vi "Actor Core.vi"(8 "error in":errorcluster, 11 "UDP_transmitter in":refnum<class "UDP_transmitter.lvclass">) -> (0 "error out":errorcluster, 3 "Actor out":refnum<class "Actor.lvclass">)   [LabVIEW 2025, in "UDP_transmitter.lvlib" / "UDP_transmitter.lvclass"]
doc: "(<B>Filename</B>: Actor Framework.lvlib:Actor.lvclass:Actor Core.vi)\n\nReceives messages to the actor, reacts to them, and initiates any error handling that may shut the actor down.\n\nDescendant classes may override this VI to append parallel tasks for the actor to complete while it handles messages. Overrides use the Call Parent Class Method node."
uses:
  UDP_transmitter.lvclass
  C:/Program Files/National Instruments/LabVIEW 2025/vi.lib/ActorFramework/Actor/Actor.lvclass
  <vilib>/ActorFramework/Actor/Actor.lvclass
  UDP_transmitter.lvclass/UDP_transmitter.ctl
  <vilib>/ActorFramework/Actor/Actor.lvclass/Actor.ctl
  <vilib>/ActorFramework/Message Enqueuer/Message Enqueuer.lvclass/Message Enqueuer.ctl
  <vilib>/ActorFramework/Message Enqueuer/Init from Existing Queue.vi
  <vilib>/ActorFramework/Message Enqueuer/Enqueue.vi
  <vilib>/ActorFramework/Stop Msg/Stop Msg.lvclass
  C:/Program Files/National Instruments/LabVIEW 2025/vi.lib/ActorFramework/Message/Message.lvclass
  <vilib>/ActorFramework/Message Priority Queue/Priority Enqueue.vi
  <vilib>/ActorFramework/Message Enqueuer/Message Enqueuer.lvclass
panel:
  in  "send_message":bool
  in  "Message":string
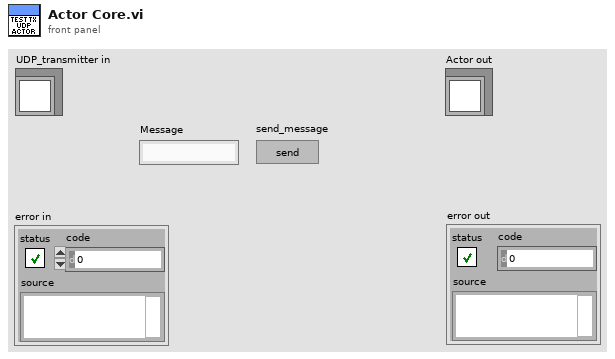
[diagram p1: front panel]
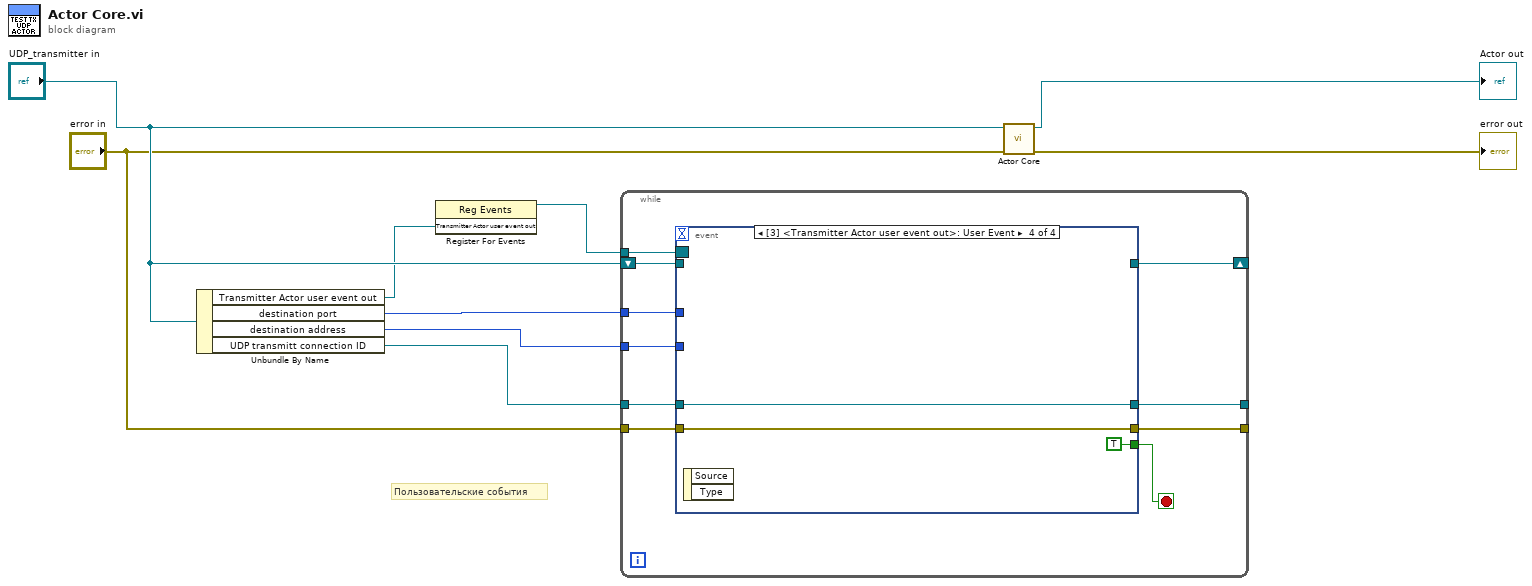
[diagram p0: block diagram]
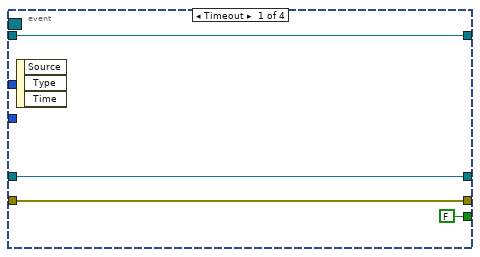
[diagram p2: hidden frame]
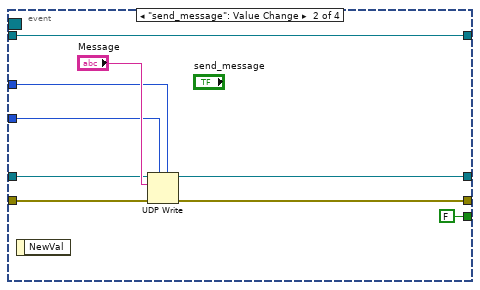
[diagram p3: hidden frame]
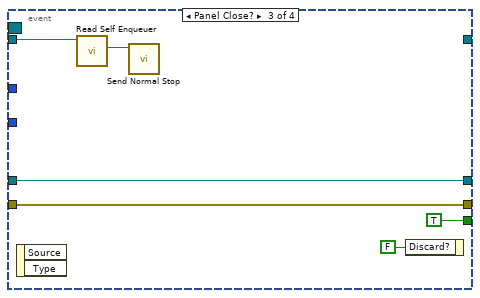
[diagram p4: hidden frame]
diagram:
  # "Пользовательские события"
  n1 = Unbundle By Name("UDP_transmitter in") -> ("Transmitter Actor user event out"=w2:refnum<user-event>, "destination port"=w4:u16, "destination address"=w3:u32, "UDP transmitt connection ID"=w6:refnum<k16>)
  n2 = register-events(w2) -> (reference out=w1:refnum<event-registration>)  [unwired: 2 in, 1 out]
  n3 = while {
    tunnel: "error in" -> [w18]
    tunnel: w6 -> [w17]
    tunnel: w3 -> [w16]
    tunnel: w4 -> [w15]
    tunnel: [w14] -> _
    tunnel: [w13] -> _
    shift-right: [w12] -> _
    shift-left: "UDP_transmitter in" -> [w19]
    tunnel: w1 -> [w10]
    stop <- w11 stop-if-true
    n4 = event shown="[3] <Transmitter Actor user event out>: User Event" {
      selector: w10 -> [_ _ _ _]
      dyn-events: _ -> [_ _ _ _]
      timeout: _ -> [_ _ _ _]
      tunnel: w19 -> [w21 w25 w36 _]
      tunnel: w18 -> [w22 w32 w37 w40]
      tunnel: w17 -> [w23 w30 w38 w41]
      tunnel: w16 -> [_ w29 _ _]
      tunnel: w15 -> [_ w28 _ _]
      tunnel: [w23 w27 w38 w41] -> w14
      tunnel: [w22 w26 w37 w40] -> w13
      tunnel: [w21 w25 _ _] -> w12
      tunnel: [FALSE FALSE TRUE TRUE] -> w11
      event Timeout {
        n5 = event-data() -> ()  [unwired: 1 in, 3 out]
      }
      event "send_message": Value Change {
        n6 = event-data() -> ()  [unwired: 1 in, 1 out]
        n7 = UDP Write(address=w29, port or service name=w28, connection ID=w30, data in="Message", 8:w32) -> (error out=w26:errorcluster, 3:w27:refnum<k16>)  [unwired: 1 in]
      }
      event Panel Close? {
        n8 = event-data() -> ()  [unwired: 1 in, 2 out]
        n9 = call <vilib>:"Read Self Enqueuer.vi"("Actor"=w36) -> ("Self Enqueuer"=w34:refnum<class "Message Enqueuer.lvclass">)  [unwired: 10 in]
        n10 = call <vilib>:"Send Normal Stop.vi"("Message Enqueuer"=w34) -> ()  [unwired: 10 in, 1 out]
        n11 = event-data("Discard?"=FALSE) -> ()  [unwired: 1 in, 1 out]
      }
      event User Event {
        n12 = event-data() -> ()  [unwired: 1 in, 2 out]
      }
    }
  }
  n13 = call-parent "Actor Core.vi"("error in"="error in", "Actor in"="UDP_transmitter in") -> ("error out"=→"error out":errorcluster, "Actor out"=→"Actor out":refnum<class "Actor.lvclass">)  [unwired: 8 in]
